vi "Test Flatten.vi"() -> ()   [LabVIEW 2021]
uses:
  ChannelRegistrar/typedef/Datatype CAN.ctl
  ChannelCommon/typedef/FIFO Header.ctl
  CIFFifoCAN.lvclass
  CIFFifoCAN.lvclass/CIFFifoCAN.ctl
  CIFFIFO/CIFfifo.lvclass/CIFfifo.ctl
  CIFFIFO/Utilities/Update Header.vi
  ChannelCommon/Utilities/Flatten Header.vi
  SubVIs/Flatten.vi/e2488641-f297-4923-bbd0-3c2628a14485.vi
  CIFFIFO/Accessors/Write T0.vi
  CIFFIFO/Accessors/Write T_Out.vi
  CIFFIFO/Accessors/Write Payload Length.vi
  CIFFIFO/Accessors/Read Header.vi
  CIFFIFO/Accessors/Write Header.vi
  CIFFIFO/Accessors/Write Timeout.vi
  ChannelCommon/Utilities/Unflatten Header.vi
  CIFUtilities/CIFClocks/SubVIs/Add Error.vi
  SubVIs/Flatten.vi/e2488641-f297-4923-bbd0-3c2628a14485.vi/c28b0ead-42ad-4072-80a2-aca7f2bd7ce3.vi
  CIFCore/Common/Utilities/Append Error Location.vi
  ChannelCommon/Utilities/Update Time.vi
  ChannelRegistrar/ChannelRegistrar.lvlib
  ChannelCommon/ChannelCommon.lvlib
panel:
  out "Header":T1={"Length"=52, "T0"=321, "T_Out"=123, "T_Tx"=1724093393726059437, "Ctr"=1}
  out "Data 2":T2={"payload"=[0, 0, 0, 0, 0, 0, 2, 51], "identifier"=291} {"payload" format="%x"; "identifier" format="%x"}
  in  "T_Out":u64=123
  in  "T0":u64=321
  in  "Data":T2={"payload"=[0, 0, 0, 0, 0, 0, 2, 51], "identifier"=291} {"payload" format="%x"; "identifier" format="%x"}
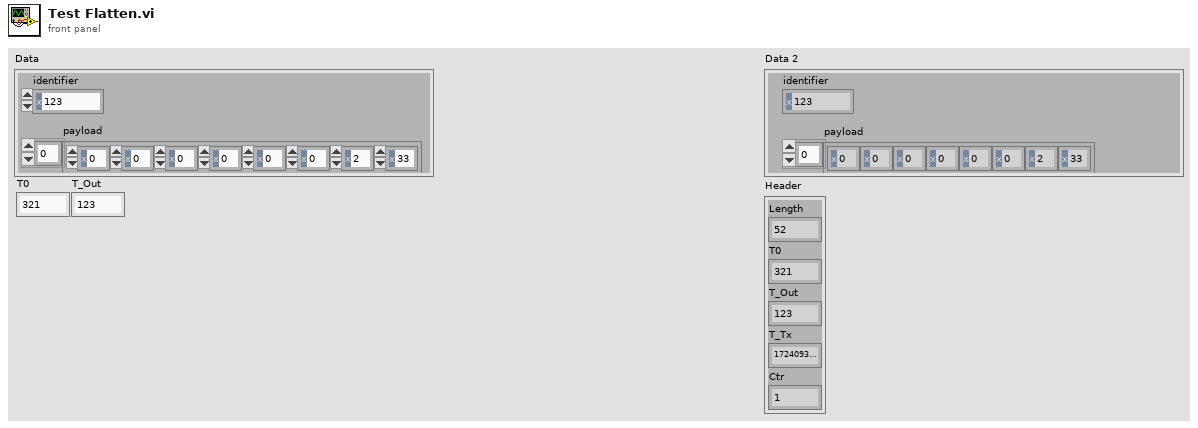
[diagram p1: front panel]
types:
  T1 = typedef "ChannelCommon.lvlib/FIFO Header.ctl" = cluster{"Length":u64, "T0":u64, "T_Out":u64, "T_Tx":u64, "Ctr":u64}
  T2 = typedef "ChannelRegistrar.lvlib/Datatype CAN.ctl" = cluster{"payload":u8[], "identifier":u32}
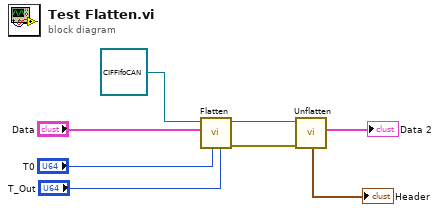
[diagram p0: block diagram]
diagram:
  n1 = call "Flatten.vi"("T_Out"="T_Out", "T0"="T0", "Data"="Data", "CIFTag in"=refnum<class "CIFFifoCAN.lvclass"> refnum) -> ("error out"=w7:errorcluster, "CIFTag out"=w8:refnum<class "CIFFifoCAN.lvclass">)  [unwired: 6 in]
  n2 = call "Unflatten.vi"("error in (no error)"=w7, "CIFFifoCAN in"=w8) -> ("Data"=→"Data 2":T2, "Header"=→"Header":T1)  [unwired: 6 in, 2 out]
